vi "setAxisGrid.vi"(7 "Grids":T1, 9 "Axis":string(combo)="x", 11 "String in":string) -> (1 "Axis out":string(combo)="x", 2 "command":string, 3 "String out":string)   [LabVIEW 2012]
uses:
  grids.ctl
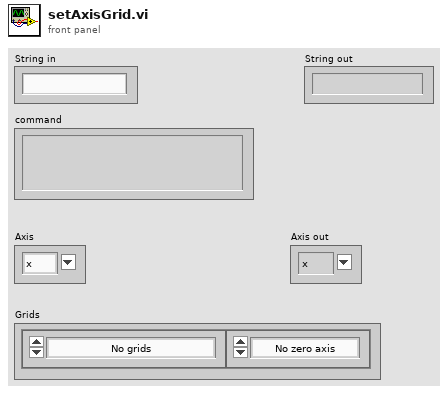
[diagram p1: front panel]
types:
  T1 = typedef "grids.ctl" = cluster{"Gridlines":enum16{"No grids", "Major grid", "Minor grid", "Major and Minor grids"}, "Zeroaxis":enum16{"No zero axis", "Show zero axis"}}
  T2 = enum16{"No grids", "Major grid", "Minor grid", "Major and Minor grids"}
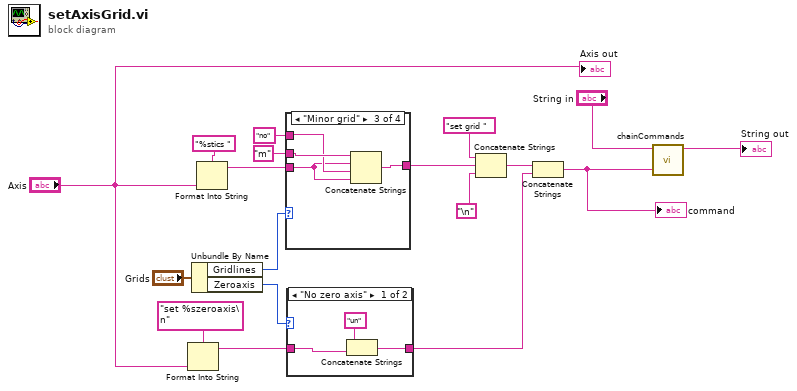
[diagram p0: block diagram]
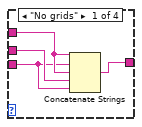
[diagram p3: hidden frame]
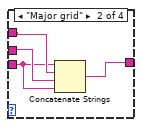
[diagram p4: hidden frame]
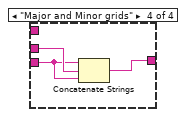
[diagram p5: hidden frame]
diagram:
  n1 = Format Into String(format string="set %szeroaxis\n", "Axis") -> (resulting string=w1:string)  [unwired: 2 in, 1 out]
  n2 = Unbundle By Name("Grids") -> ("Gridlines"=w11:T2, "Zeroaxis"=w10:enum16{"No zero axis", "Show zero axis"})
  n3 = Format Into String(format string="%stics ", "Axis") -> (resulting string=w7:string)  [unwired: 2 in, 1 out]
  n4 = case shown="\"Minor grid\"" w11 {
    tunnel: [w22 w26 w30 w31] -> w18
    tunnel: w7 -> [w19 w23 w27 w32]
    tunnel: "no" ("format string") -> [w21 w25 w28 _]
    tunnel: "m" ("format string") -> [w20 w24 w29 w33]
    frame "No grids" {
      n5 = Concatenate Strings(w21, w19, w21, w20, w19) -> (w22:string)
    }
    frame "Major grid" {
      n6 = Concatenate Strings(w23, w25, w24, w23) -> (w26:string)
    }
    frame "Minor grid" {
      n7 = Concatenate Strings(w29, w27, w28, w27) -> (w30:string)
    }
    frame "Major and Minor grids" {
      n8 = Concatenate Strings(w32, w33, w32) -> (w31:string)
    }
  }
  n9 = case shown="\"No zero axis\"" w10 {
    tunnel: [w36 w37] -> w13
    tunnel: w1 -> [w35 w37]
    frame "No zero axis" {
      n10 = Concatenate Strings("un", w35) -> (w36:string)
    }
    frame "Show zero axis" {
    }
  }
  n11 = Concatenate Strings("set grid ", w18, "\n") -> (w15:string)
  n12 = Concatenate Strings(w15, w13) -> (w14:string)
  "command" <- w14
  n13 = call "chainCommands.vi"("Command"=w14, "StringIn"="String in") -> ("StringOut"=→"String out":string)  [unwired: 9 in]
  "Axis out" <- "Axis"
